vi "Actual Sample Mode [SM].vi"(8 "error in (no error)":errorcluster, 11 "CS++Scope":refnum<class "CS++Scope.lvclass">) -> (0 "error out":errorcluster, 2 "sample mode":i32, 3 "CS++Scope out":refnum<class "CS++Scope.lvclass">)   [LabVIEW 2013, in "CS++Scope.lvlib" / "CS++Scope.lvclass"]
doc: "This VI returns the sample mode the oscilloscope is currently using."
uses:
  CS++Scope.lvclass
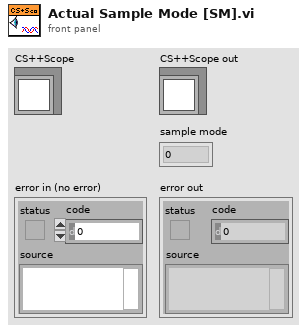
[diagram p1: front panel]
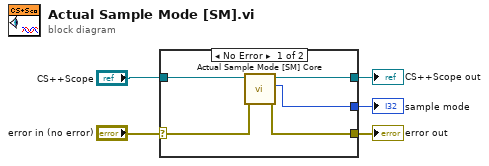
[diagram p0: block diagram]
diagram:
  n1 = case shown="No Error" "error in (no error)" {
    selector: "error in (no error)" -> [w10 w12]
    tunnel: [w9 w12] -> w4
    tunnel: [w7 w11] -> w2
    tunnel: "CS++Scope" -> [w8 w11]
    tunnel: [w6 _] -> w1
    frame No Error {
      n2 = call-dynamic "Actual Sample Mode [SM] Core.vi"("error in (no error)"=w10, "CS++Scope"=w8) -> ("error out"=w9:errorcluster, "sample mode"=w6:i32, "CS++Scope out"=w7:refnum<class "CS++Scope.lvclass">)  [unwired: 7 in]
    }
    frame Error {
    }
  }
  "error out" <- w4
  "sample mode" <- w1
  "CS++Scope out" <- w2
